vi "High Level Demo.vi"() -> ()   [LabVIEW 2011]
uses:
  Minesweeper Drawing Operation Type Def.ctl
  MineSpace.ctl
panel:
  in  "Array":T1[][](array[typedef])
  out "Minefield Picture Out":picture
  in  "column":i16
  in  "row":i16
  in  "Minesweeper Drawing Operation":T2
  in  "Stop Button":bool
  in  "Do Button":bool
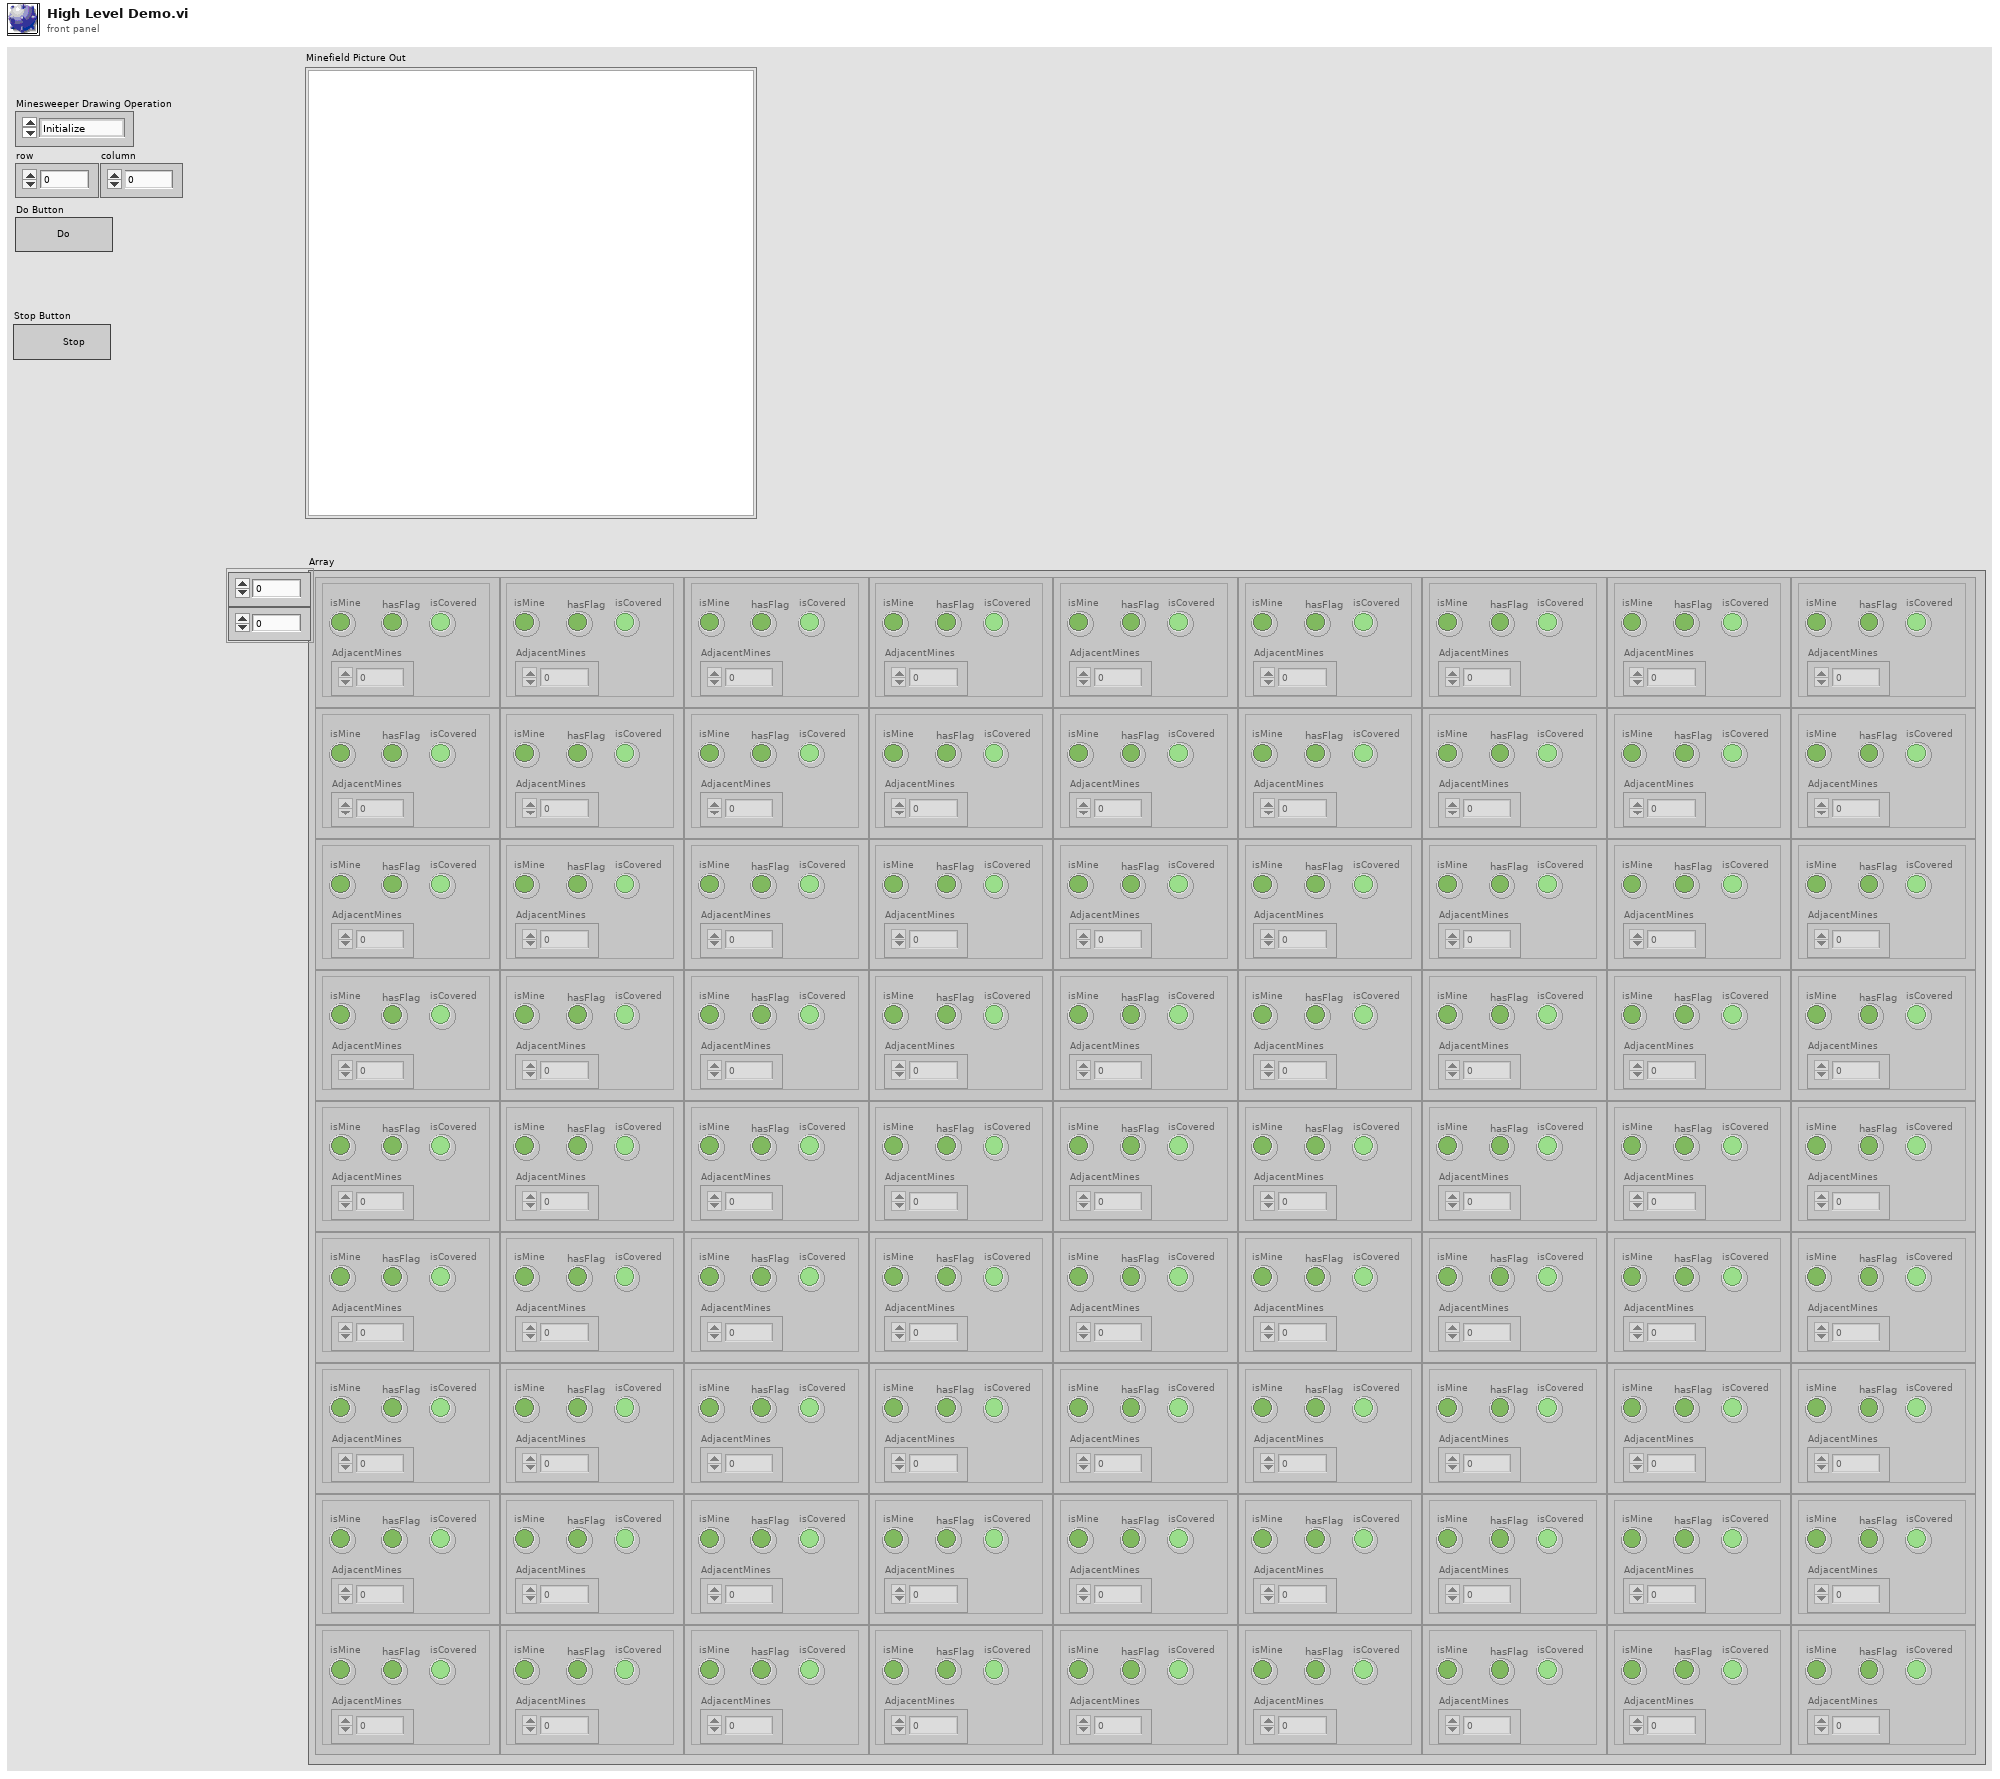
[diagram p1: front panel]
types:
  T1 = typedef "MineSpace.ctl" = cluster{"isMine":bool, "hasFlag":bool, "isCovered":bool, "AdjacentMines":u32}
  T2 = typedef "Minesweeper Drawing Operation Type Def.ctl" = enum16{"Initialize", "Uncover", "Flag", "Unflag"}
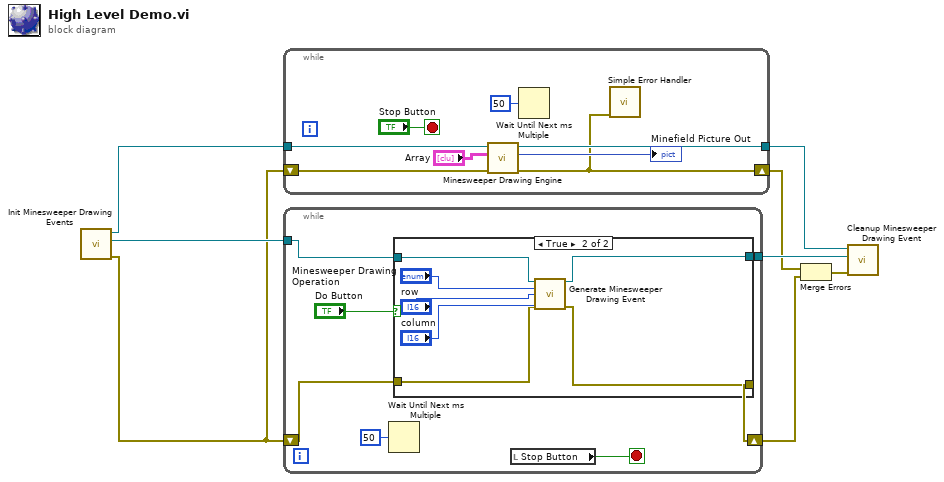
[diagram p0: block diagram]
diagram:
  n1 = call "Init Minesweeper Drawing Events.vi"() -> ("Error Out"=w4:errorcluster, "user event out"=w7:refnum<user-event>, "Event Registration Refnum"=w8:refnum<event-registration>)  [unwired: 9 in]
  n2 = while {
    tunnel: w8 -> [w16]
    tunnel: [w15] -> w5
    shift-right: [w10] -> w2
    shift-left: w4 -> [w14]
    stop <- "Stop Button" stop-if-true
    n3 = call "Minesweeper Drawing Engine.vi"("Error In"=w14, "GridData"="Array", "Event Registration Refnum"=w16) -> ("Error Out"=w10:errorcluster, "Minefield Picture Out"=→"Minefield Picture Out":picture, "Event Registration Refnum Out"=w15:refnum<event-registration>)  [unwired: 6 in]
    n4 = Wait Until Next ms Multiple(millisecond multiple=u32 50) -> ()  [unwired: 1 out]
    n5 = call <vilib>:"Simple Error Handler.vi"("error in (no error)"=w10) -> ()  [unwired: 4 in, 5 out]
  }
  n6 = while {
    tunnel: w7 -> [w19]
    tunnel: [w18] -> w6
    shift-right: [w20] -> w1
    shift-left: w4 -> [w21]
    stop <- w17 stop-if-true
    n7 = Wait Until Next ms Multiple(millisecond multiple=u32 50) -> ()  [unwired: 1 out]
    n8 = case shown="True" "Do Button" {
      tunnel: w21 -> [w24 w29]
      tunnel: [w24 w28] -> w20
      tunnel: w19 -> [w25 w27]
      tunnel: [w25 w26] -> w18
      frame False {
      }
      frame True {
        n9 = call "Generate Minesweeper Drawing Event.vi"("User Event In"=w27, "Minesweeper Drawing Operation"="Minesweeper Drawing Operation", "row"="row", "column"="column", "Error In"=w29) -> ("User Event Out"=w26:refnum<user-event>, "Error Out"=w28:errorcluster)  [unwired: 9 in]
      }
    }
    n10 = local read "Stop Button"() -> (w17:bool)
  }
  n11 = Merge Errors(w2, w1) -> (w3:errorcluster)
  n12 = call "Cleanup Minesweeper Drawing Event.vi"("Error In"=w3, "user event"=w6, "Event Registration Refnum"=w5) -> ()  [unwired: 8 in, 1 out]
